vi "Simple Lift.vi"(11 "Y axis":dbl format="%_3g") -> (3 "Lift Output":dbl)   [LabVIEW 2017]
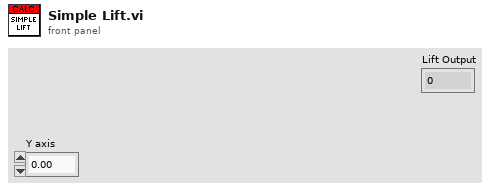
[diagram p1: front panel]
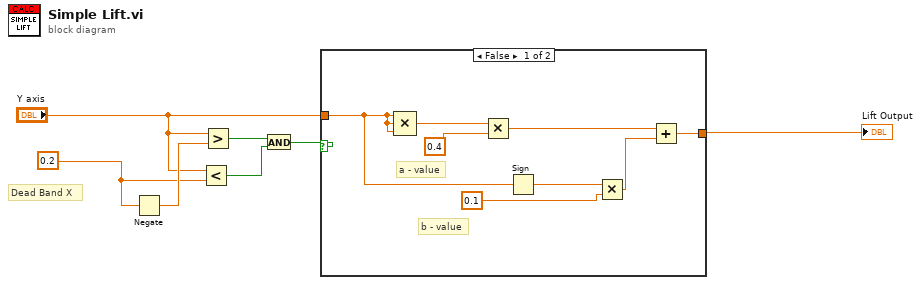
[diagram p0: block diagram]
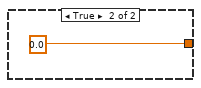
[diagram p2: hidden frame]
diagram:
  w2 = 0.2
  # "Dead Band X"
  n1 = Negate(x=w2) -> (-x=w5:dbl)
  n2 = Less?(x="Y axis", y=w2) -> (x < y?=w6:bool)
  n3 = Greater?(x="Y axis", y=w5) -> (0:w7:bool)
  n4 = And(x=w7, y=w6) -> (x .and. y?=w4:bool)
  n5 = case shown="False" w4 {
    tunnel: "Y axis" -> [w9 _]
    tunnel: [w8 0.0] -> w1
    frame False {
      # "a - value"
      # "b - value"
      n6 = Compound Arithmetic op=MULTIPLY(w9, w9, w9) -> (w12:dbl)
      n7 = Multiply(x=w12, y=0.4) -> (x*y=w13:dbl)
      n8 = Sign(1:w9) -> (0:w15:dbl)
      n9 = Multiply(x=w15, y=0.1) -> (x*y=w14:dbl)
      n10 = Add(x=w13, y=w14) -> (x+y=w8:dbl)
    }
    frame True {
    }
  }
  "Lift Output" <- w1
